vi "Init.vi"(8 "error in (no error)":errorcluster) -> (0 "error out":errorcluster, 3 "Channel DVR":refnum<data-value>)   [LabVIEW 2020, in "G-Audio.lvlib" / "Channel.lvclass"]
uses:
  Channel.lvclass
  Controls/Channel State.ctl
  Mixer/Controls/Mixer Audio Data Type.ctl
  Channel.lvclass/Channel.ctl
  Mixer/Mixer.lvclass
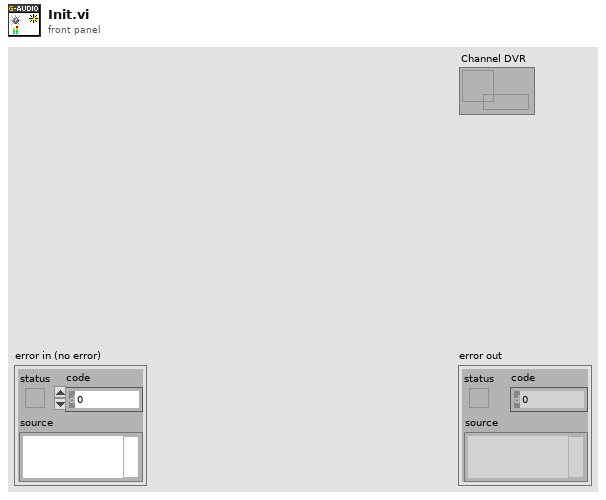
[diagram p1: front panel]
types:
  T1 = typedef "G-Audio.lvlib/Mixer.lvclass/Mixer Audio Data Type.ctl" = i16[][]
  T2 = typedef "G-Audio.lvlib/Channel.lvclass/Channel State.ctl" = enum16{"Empty", "Loading", "Stopped", "Paused", "Playing", "Retrigger"}
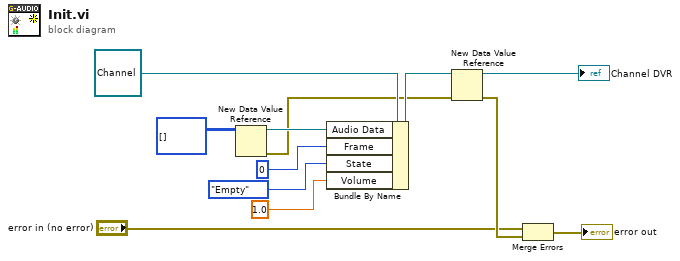
[diagram p0: block diagram]
diagram:
  n1 = New Data Value Reference(data value=T1 [] ("Audio Data")) -> (data value reference=w8:refnum<data-value>, error out=w4:errorcluster)  [unwired: 1 in]
  n2 = Bundle By Name(cluster=refnum<class "Channel.lvclass"> refnum ("G-Audio.lvlib:Channel.lvclass"), "Audio Data"=w8, "Frame"=u64 0 ("data value"), "State"=Channel_State."Empty", "Volume"=sgl 1.0 ("data value")) -> (w10:refnum<class "Channel.lvclass">)
  n3 = New Data Value Reference(data value=w10, error in=w4) -> (data value reference=→"Channel DVR":refnum<data-value>, error out=w3:errorcluster)
  n4 = Merge Errors("error in (no error)", w3) -> (→"error out":errorcluster)
